vi "STM_Server_OO.vi"() -> ()   [LabVIEW 2016, in "RemoteControl.STM.lvclass"]
uses:
  RemoteControl.STM.lvclass
  RemoteControl/Typedefs/PrivateEvents--RemoteControl.Configure.ctl
  RemoteControl/RemoteControl.lvclass
panel:
  in  "Configure":T1={"address"="", "Port"=6341, "AllowedRemote"="", "Commands"=[]}
  out "server":i32
  out "monitor":i32
  in  "Allowed Commands":T2(ring)
  in  "stop":bool
  out "error out":errorcluster
  # "SERVER  (INSTRUMENT)"
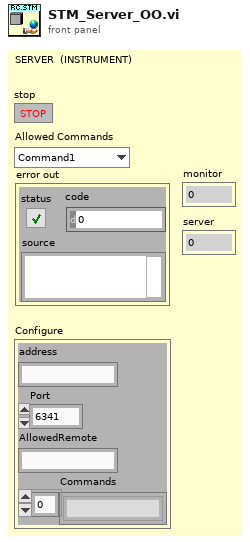
[diagram p1: front panel]
types:
  T1 = typedef "RemoteControl.lvclass/PrivateEvents--RemoteControl.Configure.ctl" = cluster{"address":string, "Port":u16, "AllowedRemote":string, "Commands":string[]}
  T2 = enum16{"Command1", "Command2", "Command3", "Command4", "HELP", "ACK", "CLOSE"}
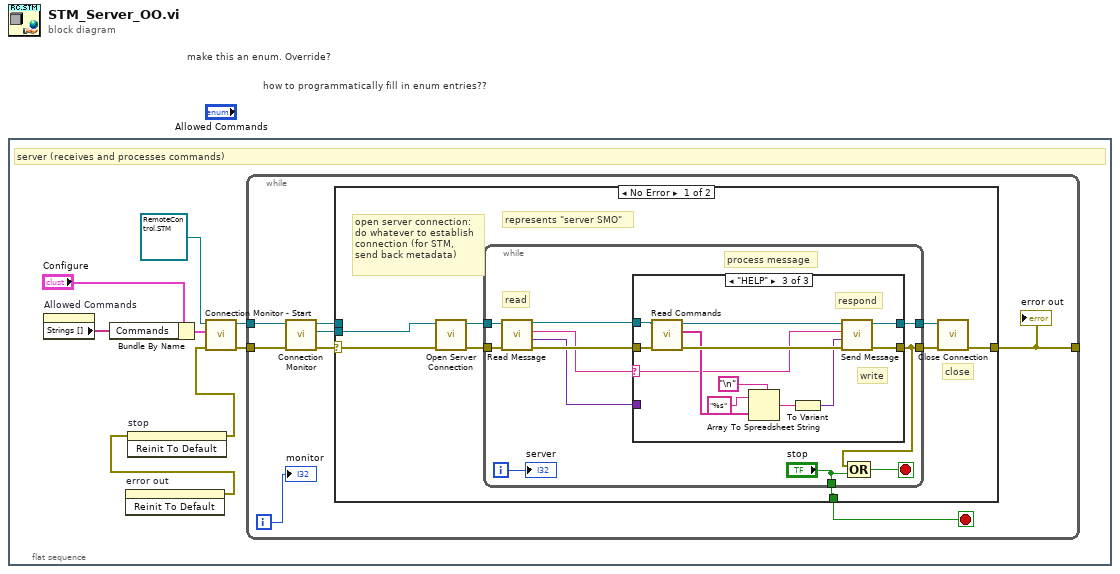
[diagram p0: block diagram]
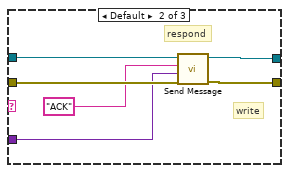
[diagram p3: hidden frame]
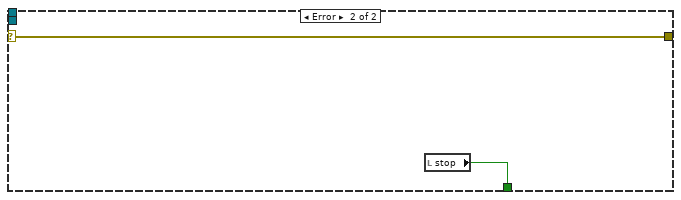
[diagram p4: hidden frame]
diagram:
  # "how to programmatically fill in enum entries??"
  # "make this an enum. Override?"
  n1 = flat-sequence {
    frame #0 {
      # "server (receives and processes commands)"
      n2 = property on="Allowed Commands" class="Enum (strict)"() -> ("Strings []"=w4:string[])  [unwired: 2 in, 2 out]
      n3 = Bundle By Name(cluster="Configure", "Commands"=w4) -> (w3:T1)
      n4 = invoke on="error out" class="Clust (strict)" method="Reinit To Default"() -> (error out=w2:errorcluster)  [unwired: 3 in, 2 out]
      n5 = invoke on="stop" class="Bool (strict)" method="Reinit To Default"(error in=w2) -> (error out=w8:errorcluster)  [unwired: 2 in, 2 out]
      n6 = call-dynamic "Connection Monitor - Start.vi"("error in (no error)"=w8, "Configure"=w3, "RemoteControl.STM in"=refnum<class "RemoteControl.STM.lvclass"> refnum ("RemoteControl.STM.lvclass")) -> ("error out"=w7:errorcluster, "RemoteControl.STM out"=w6:refnum<class "RemoteControl.STM.lvclass">)  [unwired: 7 in]
      n7 = while {
        tunnel: [w9] -> _
        tunnel: w7 -> [w13]
        tunnel: w6 -> [w12]
        i -> [w15]
        stop <- w16 stop-if-true
        n8 = call-dynamic "Connection Monitor.vi"("error in (no error)"=w13, "RemoteControl.STM in"=w12) -> ("error out"=w14:errorcluster, "Server out"=w11:refnum<class "RemoteControl.lvclass">, "RemoteControl.STM out"=w10:refnum<class "RemoteControl.STM.lvclass">)  [unwired: 7 in]
        n9 = case shown="No Error" w14 {
          selector: w14 -> [w23 w56]
          tunnel: [w24 w57] -> w16
          tunnel: [w18 w56] -> w9
          tunnel: w11 -> [w17 _]
          tunnel: w10 -> [_ _]
          frame No Error {
            # "represents \"server SMO\""
            # "close"
            # "open server connection:\ndo whatever to establish\nconnection (for STM,\nsend back metadata)"
            n10 = call-dynamic "Open Server Connection.vi"("error in (no error)"=w23, "RemoteControl in"=w17) -> ("error out"=w22:errorcluster, "RemoteControl out"=w21:refnum<class "RemoteControl.lvclass">)  [unwired: 8 in]
            n11 = while {
              tunnel: w22 -> [w34]
              tunnel: [w28] -> w19
              tunnel: [w29] -> w20
              tunnel: ["stop"] -> w24
              tunnel: w21 -> [w33]
              i -> [w27]
              stop <- w32 stop-if-true
              # "read"
              # "process message"
              n12 = call-dynamic "Read Message.vi"("error in (no error)"=w34, "RemoteControl in"=w33) -> ("error out"=w31:errorcluster, "Data"=w25:variant, "Command"=w26:string, "RemoteControl out"=w30:refnum<class "RemoteControl.lvclass">)  [unwired: 5 in, 1 out]
              n13 = case shown="\"HELP\"" w26 {
                selector: w26 -> [_ _ w46]
                tunnel: w31 -> [w37 w43 w50]
                tunnel: w30 -> [w36 w42 w51]
                tunnel: [w37 w41 w52] -> w28
                tunnel: [w36 w40 w55] -> w29
                tunnel: w25 -> [_ w38 _]
                frame "" {
                }
                frame Default {
                  # "respond"
                  # "write"
                  n14 = call-dynamic "Send Message.vi"("error in (no error)"=w43, "Data"=w38, "Command"="ACK", "RemoteControl in"=w42) -> ("error out"=w41:errorcluster, "RemoteControl out"=w40:refnum<class "RemoteControl.lvclass">)  [unwired: 6 in]
                }
                frame "HELP" {
                  # "respond"
                  # "write"
                  n15 = call-dynamic "Read Commands.vi"("error in (no error)"=w50, "RemoteControl in"=w51) -> ("error out"=w49:errorcluster, "Commands"=w47:string[], "RemoteControl out"=w48:refnum<class "RemoteControl.lvclass">)  [unwired: 7 in]
                  n16 = Array To Spreadsheet String(delimiter (Tab)="\n", array=w47, 3:"%s" ("format string")) -> (spreadsheet string=w45:string)
                  n17 = To Variant(anything=w45) -> (Variant=w44:variant)
                  n18 = call-dynamic "Send Message.vi"("error in (no error)"=w49, "Data"=w44, "Command"=w46, "RemoteControl in"=w48) -> ("error out"=w52:errorcluster, "RemoteControl out"=w55:refnum<class "RemoteControl.lvclass">)  [unwired: 6 in]
                }
              }
              n19 = Compound Arithmetic op=OR(w28, "stop") -> (w32:bool)
              "server" <- w27
            }
            n20 = call-dynamic "Close Connection.vi"("error in (no error)"=w19, "RemoteControl in"=w20) -> ("error out"=w18:errorcluster)  [unwired: 8 in, 1 out]
          }
          frame Error {
            n21 = local read "stop"() -> (w57:bool)
          }
        }
        "error out" <- w9
        "monitor" <- w15
      }
    }
  }
